vi "2020-CheesyDrive.vi"(0 "Throttle":dbl(slide)=-0.0 scale=-1.0..1.0, 1 "SlowModeSettings":i32=2, 5 "Wheel":dbl(slide) scale=-1.0..1.0) -> (4 "Left PWM":dbl=0.5949513901284444, 8 "Right PWM":dbl=0.5949513901284444)   [LabVIEW 2019]
doc: "Implements CheesyDrive. CheesyDrive means that the turn joystick controls the radius of turning instead of the rate of turning. Also implements QuickStop and QuickTurn."
uses:
  Framework/Robot Global Data.vi
panel:
  in  "FasterDeaccelerate":dbl=3.0
  in  "EnableHighSensRamp":dbl=0.8 format="%#_13g"
  in  "HighSensRamp":dbl=7.0 format="%#_13g"
  in  "ArrayOfSlownesss":T1(array[cluster])=[{"MaxSpeedSlow"=1.0, "SlowRate"=5.0, "MaxTurnSlow"=1.0, "MaxTurnRateSlow"=10.0}, {"MaxSpeedSlow"=0.6, "SlowRate"=4.0, "MaxTurnSlow"=0.8, "MaxTurnRateSlow"=10.0}, {"MaxSpeedSlow"=0.4, "SlowRate"=1.0, "MaxTurnSlow"=0.55, "MaxTurnRateSlow"=10.0}]
  in  "PointsTurn":cluster{"X":dbl, "Y":dbl}[](array[cluster])=[{"X"=0.0, "Y"=0.0}, {"X"=0.04, "Y"=0.0}, {"X"=0.041, "Y"=0.01}, {"X"=1.0, "Y"=1.0}, {"X"=1.0, "Y"=1.0}]
  in  "PointsQuickTurn":cluster{"X":dbl, "Y":dbl}[](array[cluster])=[{"X"=0.0, "Y"=0.0}, {"X"=0.04, "Y"=0.0}, {"X"=0.041, "Y"=0.2}, {"X"=0.9, "Y"=0.5}, {"X"=1.0, "Y"=1.0}]
  in  "PointsThrottle":cluster{"X":dbl, "Y":dbl}[](array[cluster])=[{"X"=0.0, "Y"=0.0}, {"X"=0.04, "Y"=0.0}, {"X"=0.0251, "Y"=0.15}, {"X"=1.0, "Y"=1.0}]
  in  "CarLikeTurning":bool
  in  "QSMult":dbl=0.1
  in  "WheelNonLinearity":dbl=0.65
  in  "negInertiaScalar":dbl=3.0
  in  "alpha":dbl=0.1
  out "Waveform Chart":dbl(graph)
  in  "Sensitivty":dbl=1.0
  # "Enable to enable"
  # "normal"
  # "(for quickstop decay)"
  # "Switch"
  # "Scale"
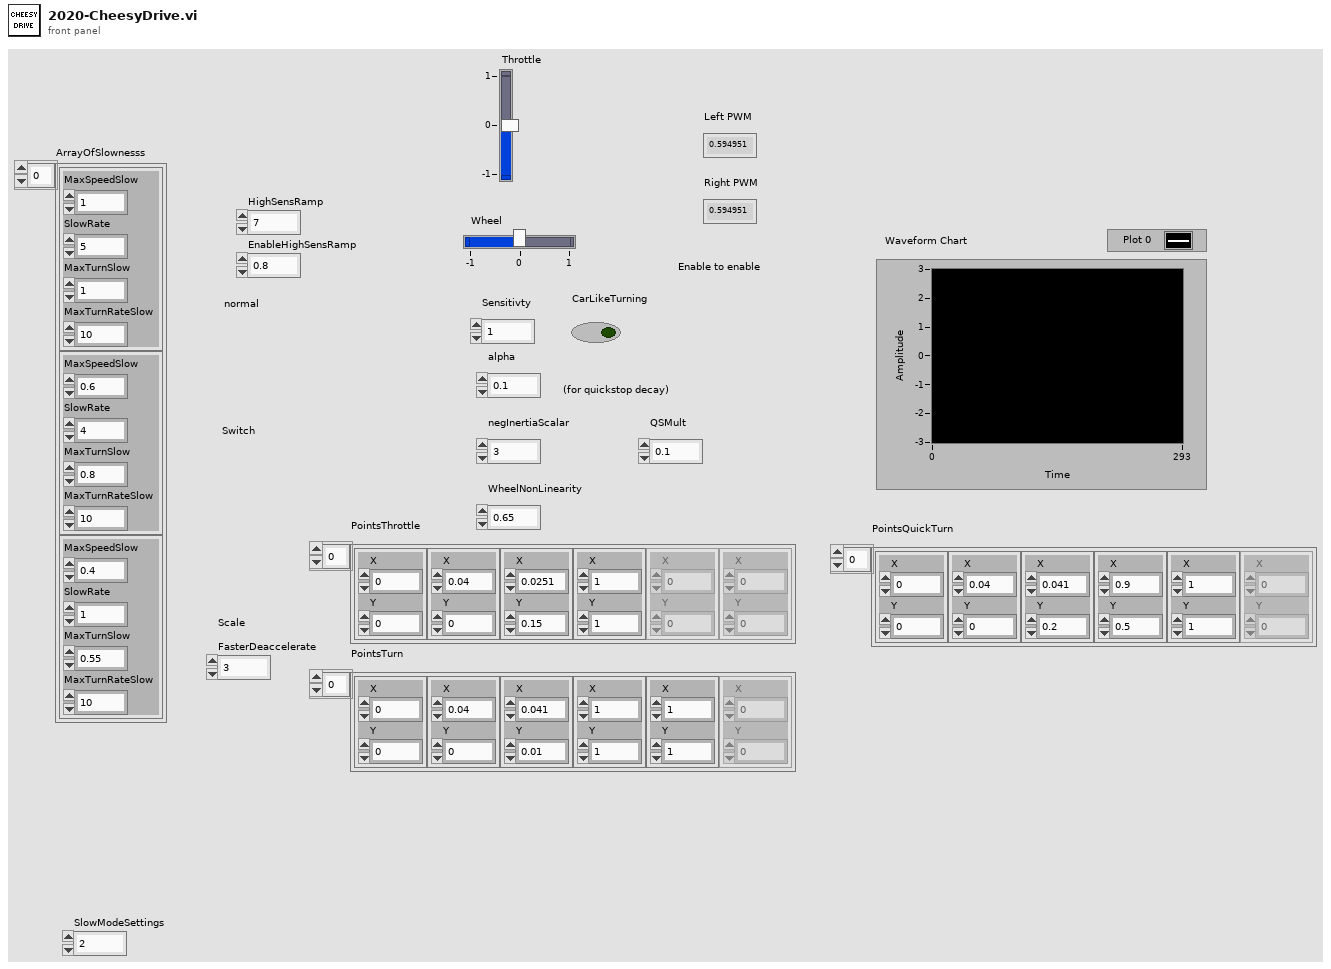
[diagram p1: front panel]
types:
  T1 = cluster{"MaxSpeedSlow":dbl, "SlowRate":dbl, "MaxTurnSlow":dbl, "MaxTurnRateSlow":dbl}[]
  T2 = cluster{"MaxSpeedSlow":dbl, "SlowRate":dbl, "MaxTurnSlow":dbl, "MaxTurnRateSlow":dbl}
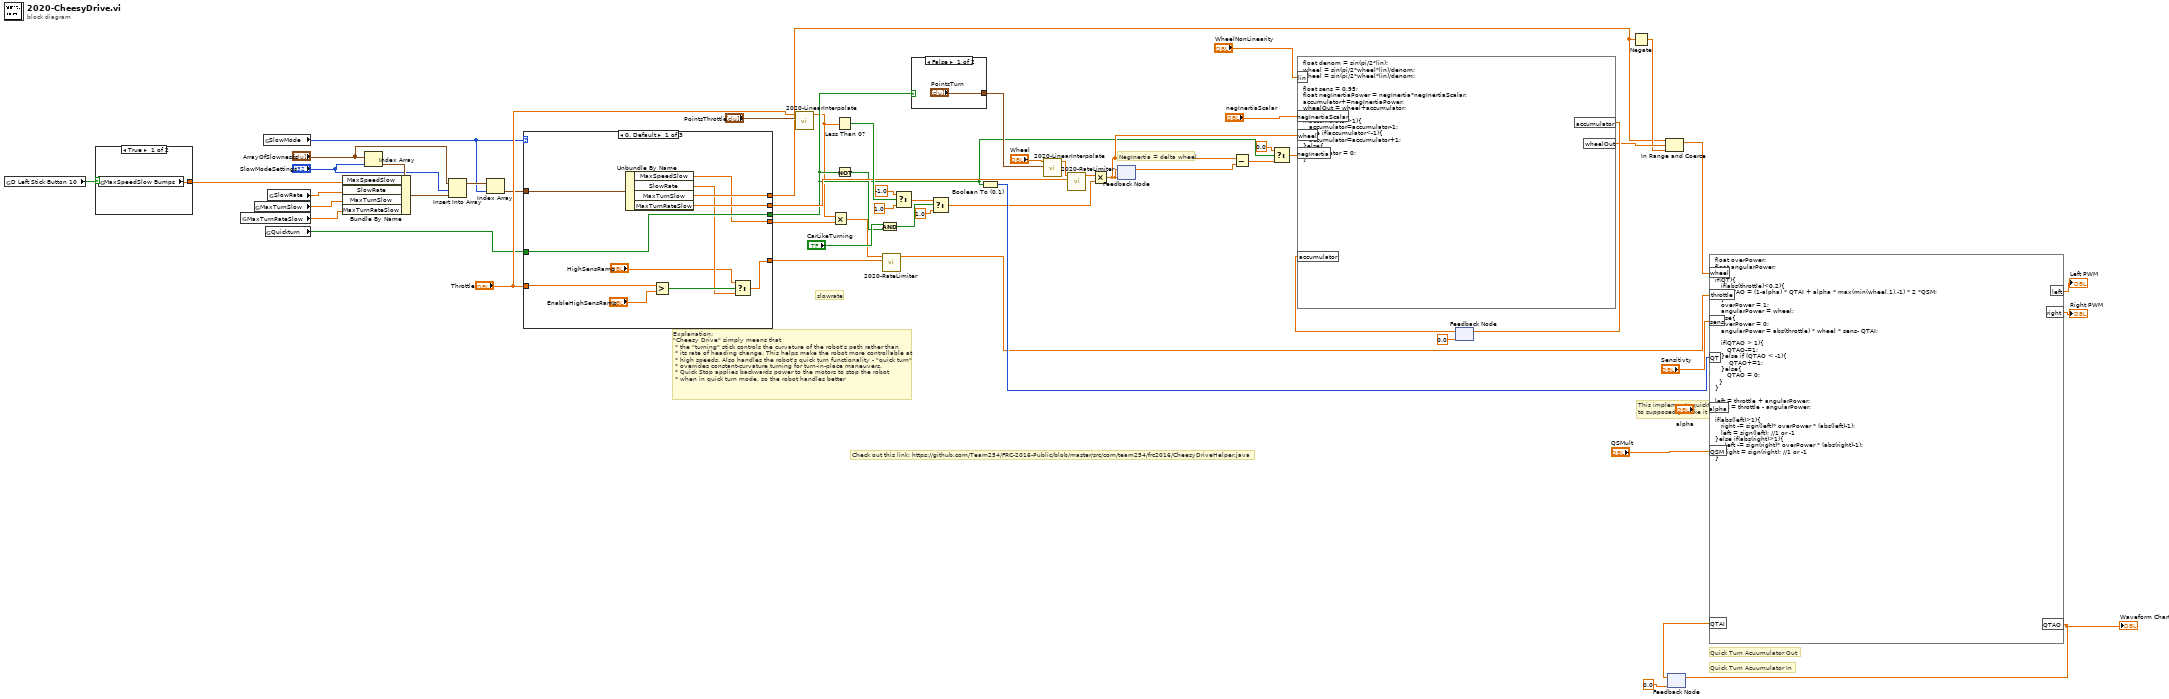
[diagram p0: block diagram]
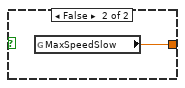
[diagram p2: hidden frame]
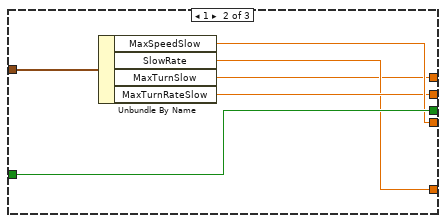
[diagram p3: hidden frame]
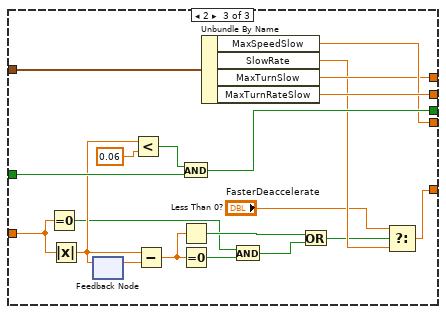
[diagram p4: hidden frame]
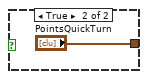
[diagram p5: hidden frame]
diagram:
  # "slowrate"
  # "This implements quickturn and also modifies wheel with a sine function\nto supposedly make it easier to drive"
  # "NegInertia = delta wheel"
  # "Explanation:\n\"Cheesy Drive\" simply means that\n * the \"turning\" stick controls the curvature of the robot's path rather than\n * its rate of heading change. This helps make the robot more controllable at\n * high speeds. Also handles the robot's quick turn functionality - \"quick turn\"\n * overrides constant-curvature turning for turn-in-place maneuvers.\n * Quick Stop applies backwards power to the motors to stop the robot\n * when in quick turn mode, so the robot handles better"
  # "Quick Turn Acuumulator Out"
  # "Quick Turn Acuumulator In"
  # "Check out this link: https://github.com/Team254/FRC-2016-Public/blob/master/src/com/team254/frc2016/CheesyDriveHelper.java"
  n1 = global read "Robot Global Data.vi" "D Left Stick Button 10"() -> (w1:bool)
  n2 = case shown="True" w1 {
    tunnel: [w59 w60] -> w7
    frame True {
      n3 = global read "Robot Global Data.vi" "MaxSpeedSlow Bumps"() -> (w59:dbl)
    }
    frame False {
      n4 = global read "Robot Global Data.vi" "MaxSpeedSlow"() -> (w60:dbl)
    }
  }
  n5 = global read "Robot Global Data.vi" "MaxTurnRateSlow"() -> (w4:dbl)
  n6 = global read "Robot Global Data.vi" "MaxTurnSlow"() -> (w5:dbl)
  n7 = global read "Robot Global Data.vi" "SlowMode"() -> (w2:u32)
  n8 = global read "Robot Global Data.vi" "Quickturn"() -> (w3:bool)
  n9 = global read "Robot Global Data.vi" "SlowRate"() -> (w6:dbl)
  n10 = Index Array(array="ArrayOfSlownesss", index="SlowModeSettings") -> (element=w13:T2)
  n11 = Bundle By Name(cluster=w13, "MaxSpeedSlow"=w7, "SlowRate"=w6, "MaxTurnSlow"=w5, "MaxTurnRateSlow"=w4) -> (w11:T2)
  n12 = Insert Into Array(array="ArrayOfSlownesss", index="SlowModeSettings", new element=w11) -> (w10:T1)
  n13 = Index Array(array=w10, index=w2) -> (element=w9:T2)
  n14 = case shown="0, Default" w2 {
    tunnel: [w62 w74 w87] -> w30
    tunnel: [w68 w76 w90] -> w14
    tunnel: [w69 w73 w89] -> w28
    tunnel: [w70 w75 w91] -> w25
    tunnel: w3 -> [w71 w77 w97]
    tunnel: [w71 w77 w94] -> w17
    tunnel: "Throttle" -> [w67 _ w84]
    tunnel: w9 -> [w61 w72 w78]
    frame 0, Default {
      n15 = Unbundle By Name(w61) -> ("MaxSpeedSlow"=w68:dbl, "SlowRate"=w64:dbl, "MaxTurnSlow"=w69:dbl, "MaxTurnRateSlow"=w70:dbl)
      n16 = Greater?(x=w67, y="EnableHighSensRamp") -> (0:w65:bool)
      n17 = Select(t="HighSensRamp", s=w65, f=w64) -> (s? t:f=w62:dbl)
    }
    frame 1 {
      n18 = Unbundle By Name(w72) -> ("MaxSpeedSlow"=w76:dbl, "SlowRate"=w74:dbl, "MaxTurnSlow"=w73:dbl, "MaxTurnRateSlow"=w75:dbl)
    }
    frame 2 {
      n19 = Equal To 0?(x=w84) -> (x = 0?=w83:bool)
      n20 = Absolute Value(x=w84) -> (abs(x)=w92:dbl)
      n21 = feedback-in #1(w92) -> ()
      n22 = feedback #1() -> (w93:dbl)  [unwired: 1 in]
      n23 = Less?(x=w92, y=0.06) -> (x < y?=w96:bool)
      n24 = Subtract(x=w92, y=w93) -> (x-y=w82:dbl)
      n25 = And(x=w96, y=w97) -> (x .and. y?=w94:bool)
      n26 = Less Than 0?(x=w82) -> (x < 0?=w85:bool)
      n27 = Equal To 0?(x=w82) -> (x = 0?=w80:bool)
      n28 = Unbundle By Name(w78) -> ("MaxSpeedSlow"=w90:dbl, "SlowRate"=w88:dbl, "MaxTurnSlow"=w89:dbl, "MaxTurnRateSlow"=w91:dbl)
      n29 = And(x=w83, y=w80) -> (x .and. y?=w81:bool)
      n30 = Or(x=w85, y=w81) -> (x .or. y?=w79:bool)
      n31 = Select(t="FasterDeaccelerate", s=w79, f=w88) -> (s? t:f=w87:dbl)
    }
  }
  n32 = call "2020-LinearInterpolate.vi"("Points"="PointsThrottle", "Value"="Throttle") -> ("Output"=w16:dbl)  [unwired: 9 in]
  n33 = Multiply(x=w16, y=w14) -> (x*y=w15:dbl)
  n34 = Less Than 0?(x=w16) -> (x < 0?=w40:bool)
  n35 = Not(x=w17) -> (.not. x?=w19:bool)
  n36 = And(x="CarLikeTurning", y=w19) -> (x .and. y?=w18:bool)
  n37 = call "2020-RateLimiter.vi"("Max dx/dt"=w30, "Input"=w15) -> ("Output"=w52:dbl)  [unwired: 9 in]
  n38 = Select(t=-1.0, s=w40, f=1.0) -> (s? t:f=w36:dbl)
  n39 = case shown="False" w17 {
    tunnel: ["PointsTurn" "PointsQuickTurn"] -> w32
    frame False {
    }
    frame True {
    }
  }
  n40 = Select(t=w36, s=w18, f=1.0) -> (s? t:f=w34:dbl)
  n41 = Boolean To (0,1)(Boolean=w17) -> (0, 1=w56:i16)
  n42 = call "2020-LinearInterpolate.vi"("Points"=w32, "Value"="Wheel") -> ("Output"=w27:dbl)  [unwired: 9 in]
  n43 = call "2020-RateLimiter.vi"("Max dx/dt"=w25, "Input"=w27) -> ("Output"=w26:dbl)  [unwired: 9 in]
  n44 = Multiply(x=w26, y=w34) -> (x*y=w37:dbl)
  n45 = feedback #2(w37) -> (w49:dbl)
  n46 = feedback-in #2(w37) -> ()
  n47 = Subtract(x=w37, y=w49) -> (x-y=w23:dbl)
  n48 = Select(t=0.0, s=w17, f=w23) -> (s? t:f=w24:dbl)
  n49 = feedback #3(0.0 ("Wheel")) -> (w48:dbl)
  n50 = formula code="float denom = sin(pi/2*lin);\nwheel = sin(pi/2*wheel*lin)/denom;\nwheel = sin(pi/2*wheel*lin)/denom;\n\nfloat sens = 0.95;\nfloat negInertiaPower = negInertia*negInertiaScalar;\naccumulator+=negInertiaPower;\nwheelOut = wheel+accumulator;\n\nif(accumulator>1){\n   accumulator=accumulator-1;\n}else if(accumulator<-1){\n   accumulator=accumulator+1;\n}else{\naccumulator = 0;\n}"("wheel"=w37, "negInertia"=w24, "accumulator"=w48, "negInertiaScalar"="negInertiaScalar", "lin"="WheelNonLinearity") -> ("accumulator"=w46:dbl, "wheelOut"=w42:dbl)
  n51 = feedback-in #3(w46) -> ()
  n52 = Negate(x=w28) -> (-x=w29:dbl)
  n53 = In Range and Coerce(upper limit=w28, x=w42, lower limit=w29) -> (coerced(x)=w43:dbl)  [unwired: 1 out]
  n54 = feedback #4(0.0 ("QTAccumulatorO")) -> (w54:dbl)
  n55 = formula code="float overPower;\nfloat angularPower;\n\nif(QT){\n   if(abs(throttle)<0.2){\n      QTAO = (1-alpha) * QTAI + alpha * max(min(wheel,1),-1) * 2 *QSM;\n   }\n   overPower = 1;\n   angularPower = wheel;\n}else{\n   overPower = 0;\n   angularPower = abs(throttle) * wheel * sens- QTAI;\n\n   if(QTAO > 1){\n      QTAO-=1;\n   }else if (QTAO < -1){\n       QTAO+=1;\n   }else{\n      QTAO = 0;\n  }\n}\n\nleft = throttle + angularPower;\nright = throttle - angularPower;\n\nif(abs(left)>1){\n   right -= sign(left)* overPower * (abs(left)-1);\n   left = sign(left); //1 or -1\n}else if(abs(right)>1){\n     left -= sign(right)* overPower * (abs(right)-1);\n     right = sign(right); //1 or -1 \n}"("wheel"=w43, "throttle"=w52, "sens"="Sensitivty", "QT"=w56, "alpha"="alpha", "QTAI"=w54, "QSM"="QSMult") -> ("left"=→"Left PWM":dbl, "right"=→"Right PWM":dbl, "QTAO"=w57:dbl)
  "Waveform Chart" <- w57
  n56 = feedback-in #4(w57) -> ()
